vi "create_report_file.vi"(8 "error in (no error)":errorcluster, 11 "UI":T1) -> (0 "error out":errorcluster, 3 "output cluster":T1)   [LabVIEW 2017]
uses:
  ui.ctl
  classes/dc_power_supply/DC_power_supply.lvclass
  classes/report/Report.lvclass
  ui_buttons.ctl
  types/boc_type.ctl
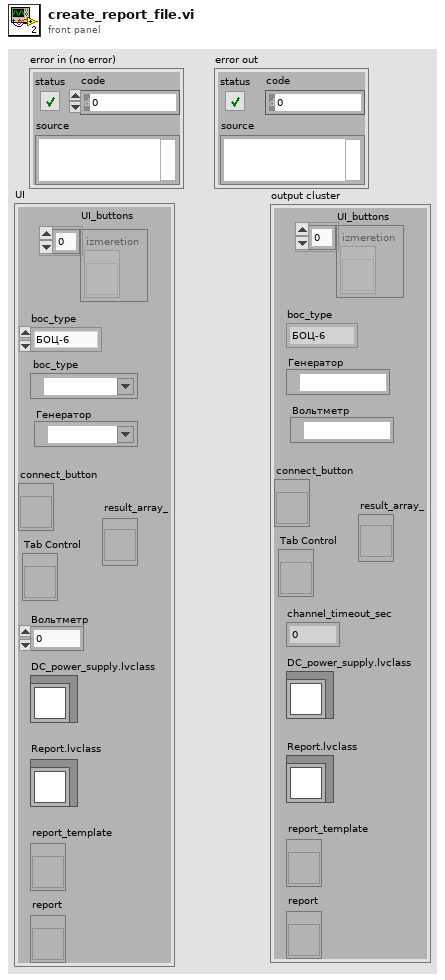
[diagram p1: front panel]
types:
  T1 = typedef "ui.ctl" = cluster{"UI_buttons":T2, "Tab Control":refnum<vi>, "connect_button":refnum<vi>, "generator":refnum<visa-resource-name>, "voltmetr":refnum<visa-resource-name>, "channel_timeout_sec":dbl, "boc_type":T3, "result_array_":refnum<vi>, "DC_power_supply.lvclass":refnum<class "DC_power_supply.lvclass">, "Report.lvclass":refnum<class "Report.lvclass">, "report_template":refnum<vi>, "report":refnum<vi>}
  T2 = typedef "ui_buttons.ctl" = refnum<vi>[]
  T3 = typedef "boc_type.ctl" = enum16{"БОЦ-6", "БОЦ-12"}
  T4 = enum16{"open", "replace", "create", "open or create", "replace or create", "replace or create with confirmation"}
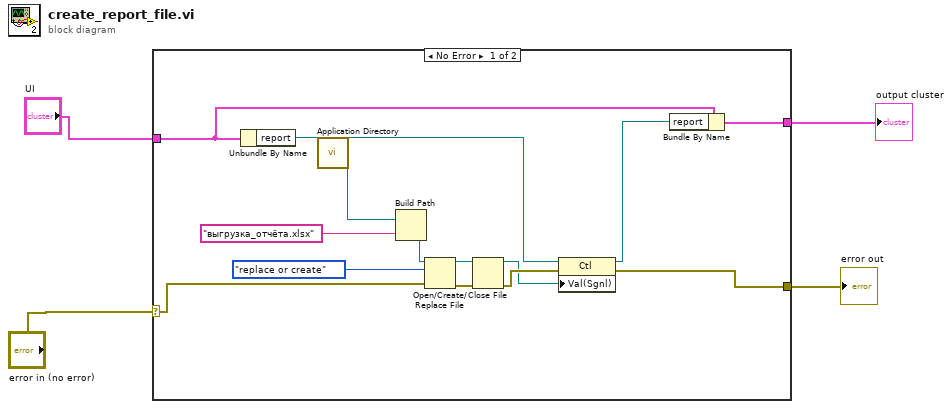
[diagram p0: block diagram]
diagram:
  n1 = case shown="No Error" "error in (no error)" {
    selector: "error in (no error)" -> [w5 w19]
    tunnel: [w14 w19] -> w4
    tunnel: "UI" -> [w8 w20]
    tunnel: [w6 w20] -> w2
    frame No Error {
      n2 = Unbundle By Name(w8) -> ("report"=w9:refnum<vi>)
      n3 = call <vilib>:"Application Directory.vi"() -> ("Application Directory"=w17:path)
      n4 = Build Path(base path=w17, name or relative path="выгрузка_отчёта.xlsx") -> (appended path=w18:path)
      n5 = Open/Create/Replace File(file path (use dialog)=w18, error in=w5, operation (0:open)=T4."replace or create") -> (refnum out=w12:refnum<file>, error out=w11:errorcluster)  [unwired: 3 in, 1 out]
      n6 = Close File(refnum=w12, error in=w11) -> (path=w13:path, error out=w15:errorcluster)
      n7 = property class="Ctl"(reference=w9, error in=w15, "Val(Sgnl)"=w13) -> (reference out=w7:refnum<vi>, error out=w14:errorcluster)
      n8 = Bundle By Name(cluster=w8, "report"=w7) -> (w6:T1)
    }
    frame Error {
    }
  }
  "error out" <- w4
  "output cluster" <- w2
